vi "Create.vi"(8 "error in (no error)":errorcluster, 10 "Config Manager":refnum<class "Config Manager.lvclass">, 11 "Group":string) -> (0 "error out":errorcluster, 3 "Pref Group out":refnum<class "Pref Group.lvclass">)   [LabVIEW 2020, in "User Prefs.lvlib" / "Pref Group.lvclass"]
uses:
  Pref Group.lvclass
  Pref Group.lvclass/Pref Group.ctl
  lv-cdm/CDM-Config/Config Manager/Config Manager.lvclass
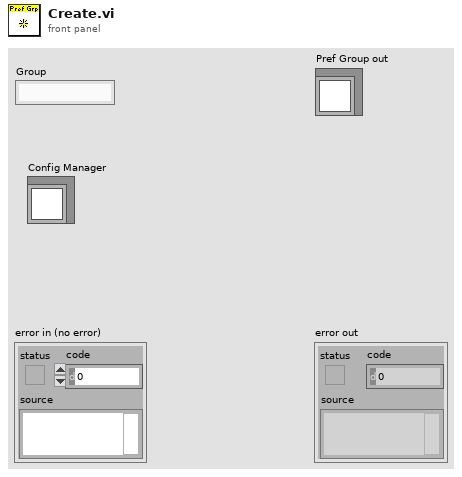
[diagram p1: front panel]
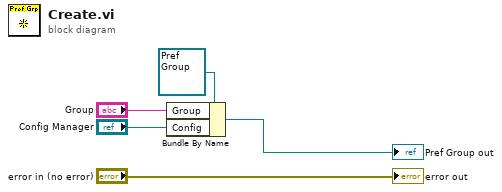
[diagram p0: block diagram]
diagram:
  n1 = Bundle By Name(cluster=refnum<class "Pref Group.lvclass"> refnum ("Pref Group in"), "Group"="Group", "Config"="Config Manager") -> (→"Pref Group out":refnum<class "Pref Group.lvclass">)
  "error out" <- "error in (no error)"
